vi "Set Logged Data Subpanel.vi"(10 "Data Logger Subpanel":refnum<vi>, 11 "Series Actor in":refnum<class "Series Actor.lvclass">) -> (3 "Series Actor out":refnum<class "Series Actor.lvclass">)   [LabVIEW 2023, in "Series Actor.lvlib" / "Series Actor.lvclass"]
uses:
  Series Actor.lvclass
  Series Actor.lvclass/Series Actor.ctl
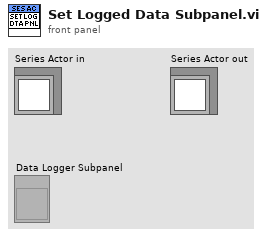
[diagram p1: front panel]
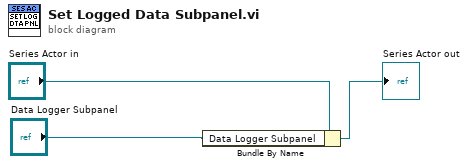
[diagram p0: block diagram]
diagram:
  n1 = Bundle By Name(cluster="Series Actor in", "Data Logger Subpanel"="Data Logger Subpanel") -> (→"Series Actor out":refnum<class "Series Actor.lvclass">)
